vi "GUI_Camera_FFT.vi"() -> ()   [LabVIEW 2020]
uses:
  Shared/GUI_Template/GUI_master/tcp_new_data_event.ctl
  Shared/GUI_Template/GUI_master/tcp new data cluster.ctl
panel:
  out "tcp data event":T1
  in  "Refresh Button":bool
  in  "Select device":string(combo)="PL1-PresCtl"
  in  "stop":bool
  in  "triggermode::1":bool caption="Blank Button"
  in  "exposure::1":dbl=0.001 caption="Exposure" min=0.0001 max=1.0 format="%_4p"
  in  "GUIdevice 1":string="TS-ChromexCam"
  out "image::1":T2(plugin-control) caption="image for joost"
  in  "insert tag":bool=TRUE
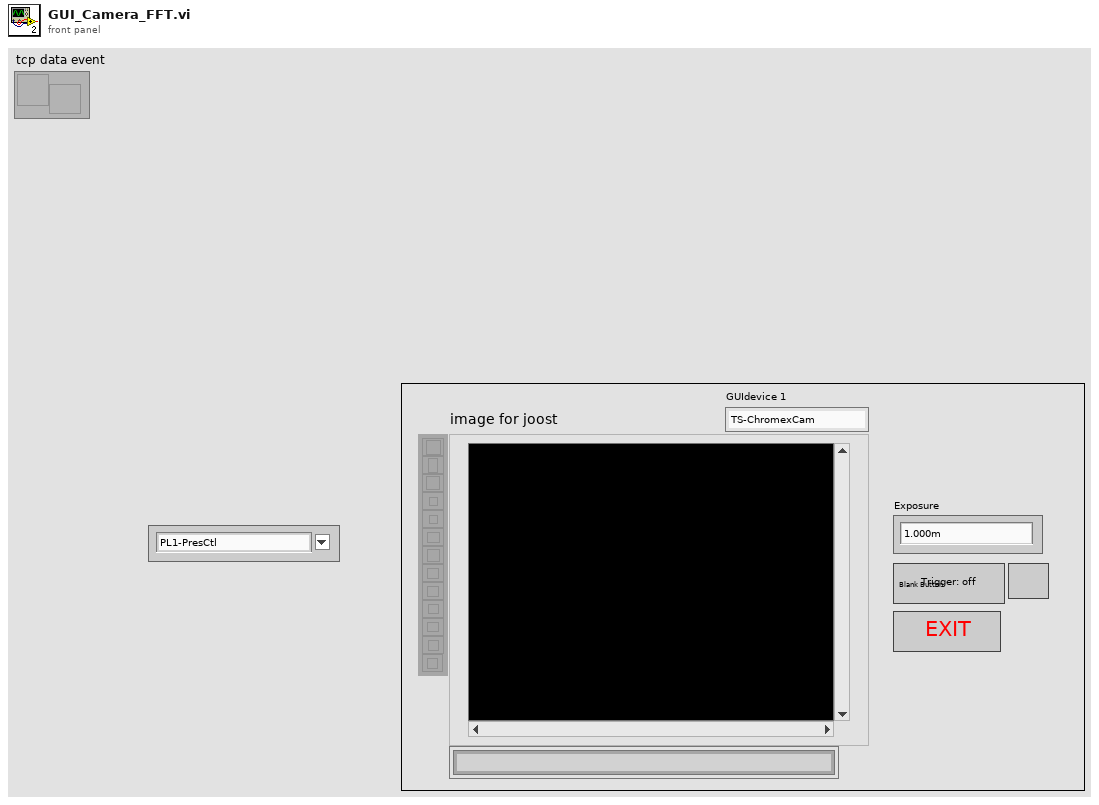
[diagram p1: front panel]
types:
  T1 = typedef "tcp_new_data_event.ctl" = refnum<user-event>
  T2 = typedef "IMAQ Image.ctl" = refnum<image>
  T3 = typedef "Image Type" = u32
  T4 = enum32{"invalid app kind", "Development System", "Run Time System", "Student Edition", "Embedded LabVIEW", "Evaluation", "Custom"}
  T5 = typedef "tcp new data cluster.ctl" = cluster{"EventEnum":enum16{"new data", "connection status update"}, "Device name":string}
  T6 = enum32{"Invalid", "Standard", "Closed", "Hidden", "Minimized", "Maximized"}
  T7 = cluster{"Core":cluster{"Current VI Reference":refnum<vi>, "Close Panel on Exit?":bool}, "Your Boolean data":bool, "Your string data":string, "SuperGUI":cluster{"STOP queue":refnum<queue>, "SuperGUI ref":refnum<vi>}}
  T8 = cluster{"STOP queue":refnum<queue>, "SuperGUI ref":refnum<vi>}
  T9 = cluster{"Current VI Reference":refnum<vi>, "Close Panel on Exit?":bool}
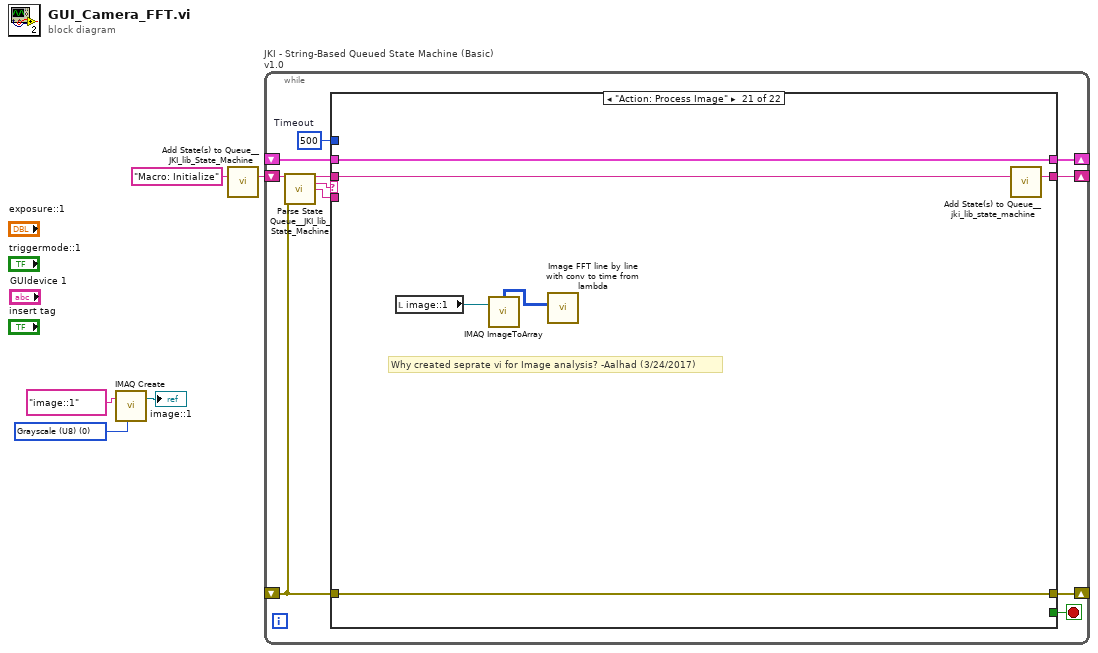
[diagram p0: block diagram]
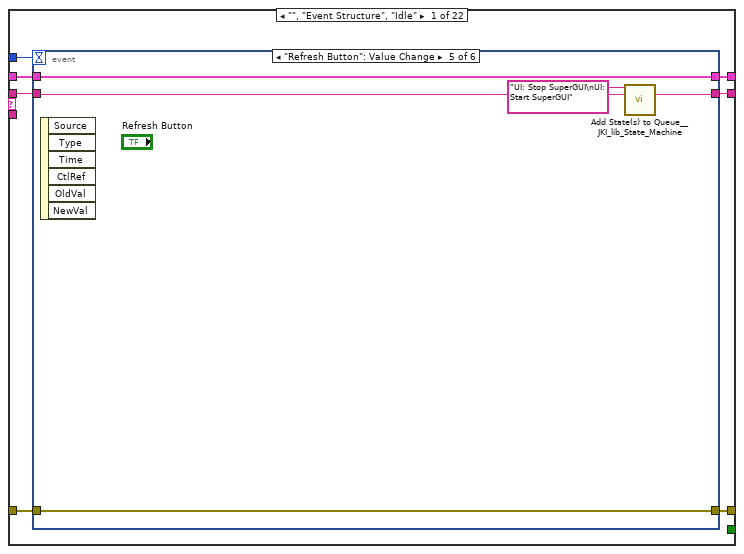
[diagram p2: hidden frame]
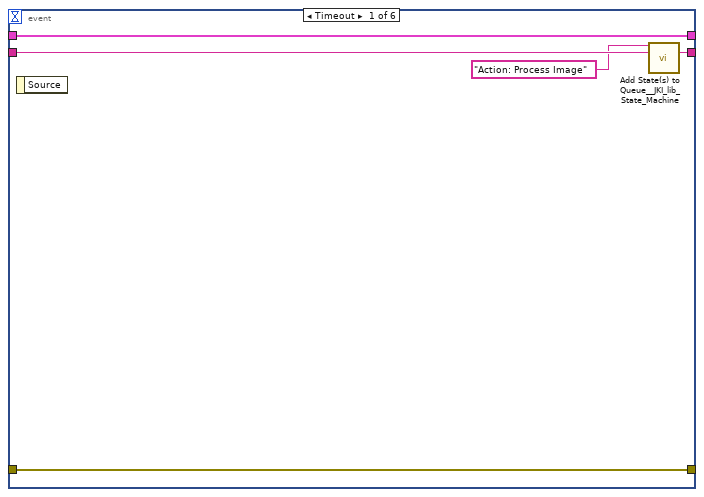
[diagram p3: hidden frame]
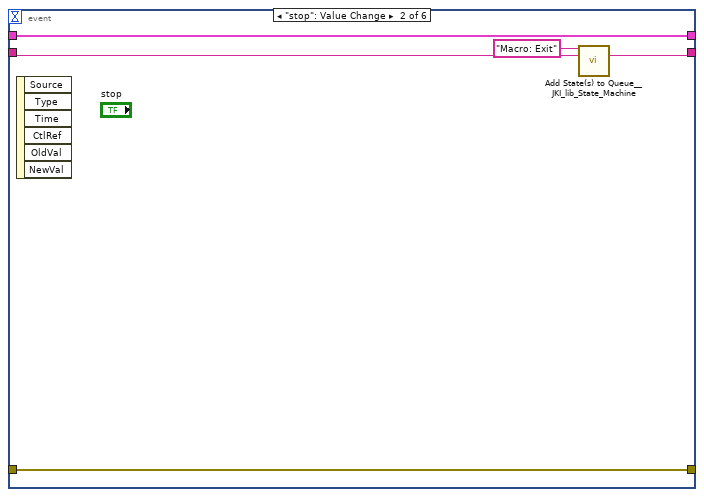
[diagram p4: hidden frame]
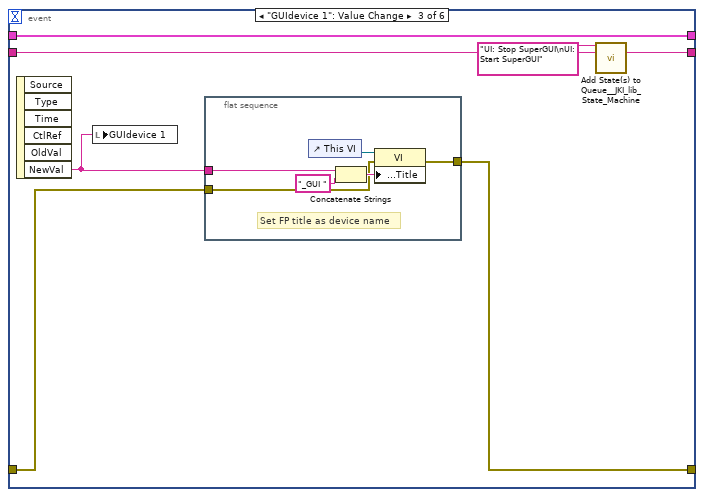
[diagram p5: hidden frame]
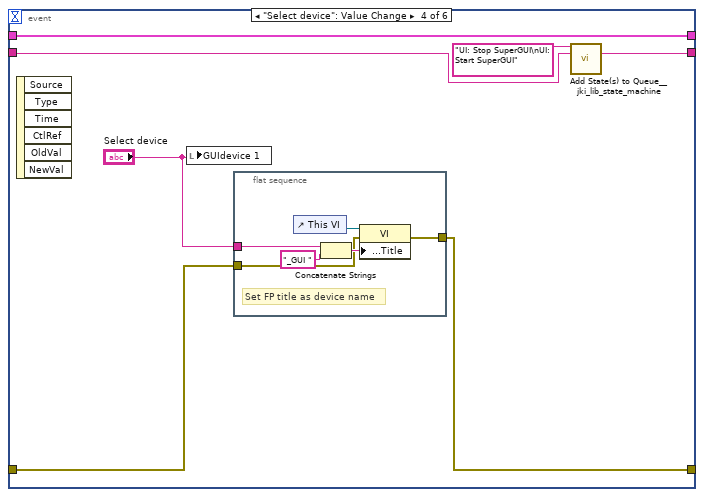
[diagram p6: hidden frame]
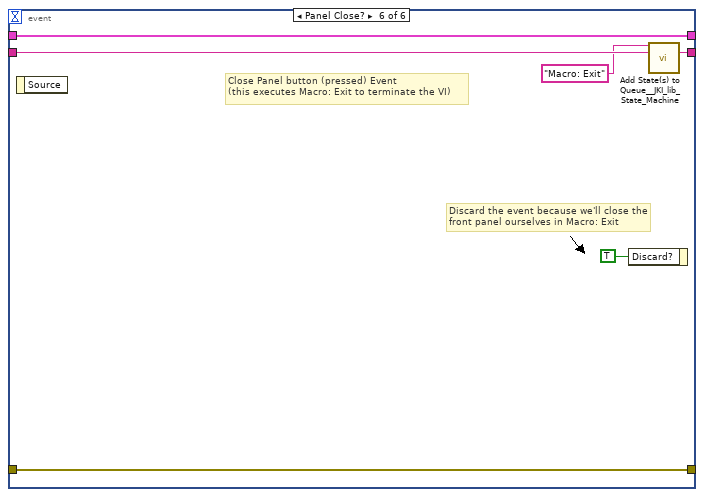
[diagram p7: hidden frame]
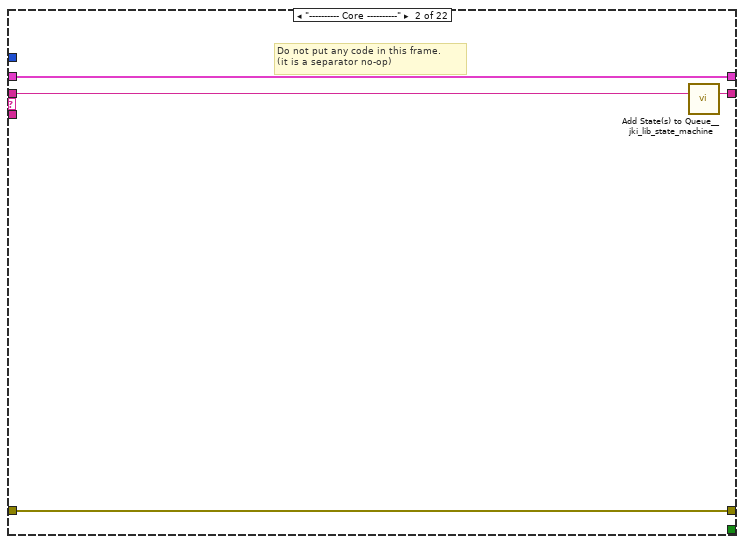
[diagram p8: hidden frame]
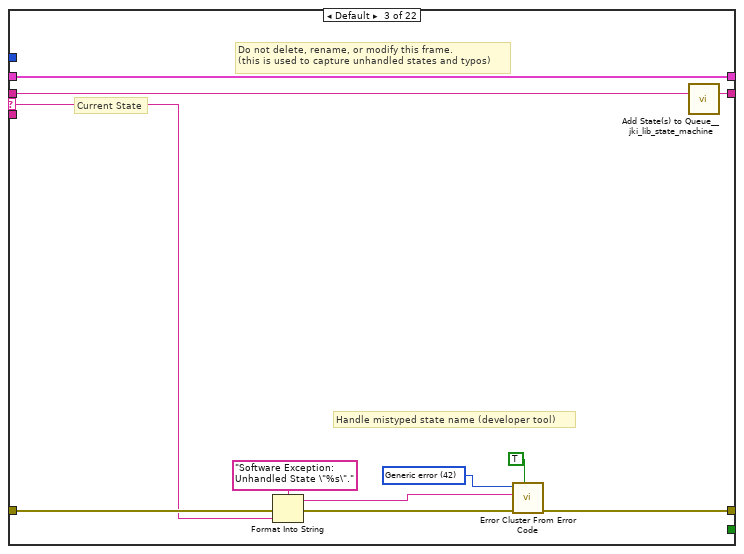
[diagram p9: hidden frame]
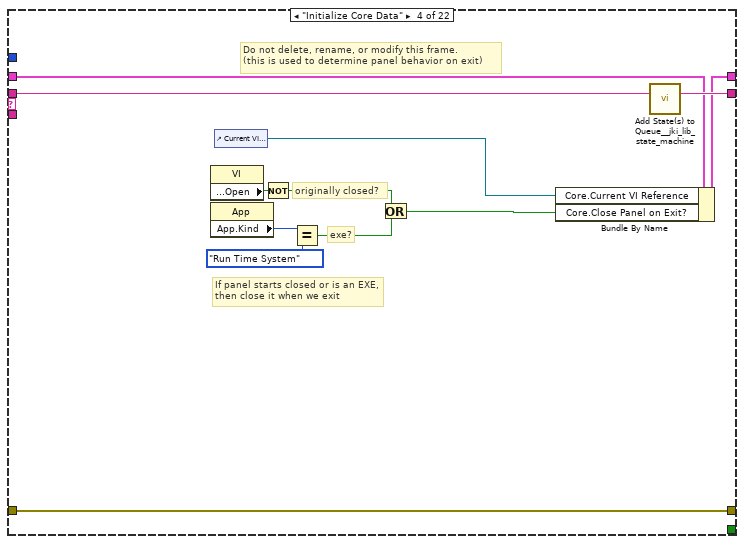
[diagram p10: hidden frame]
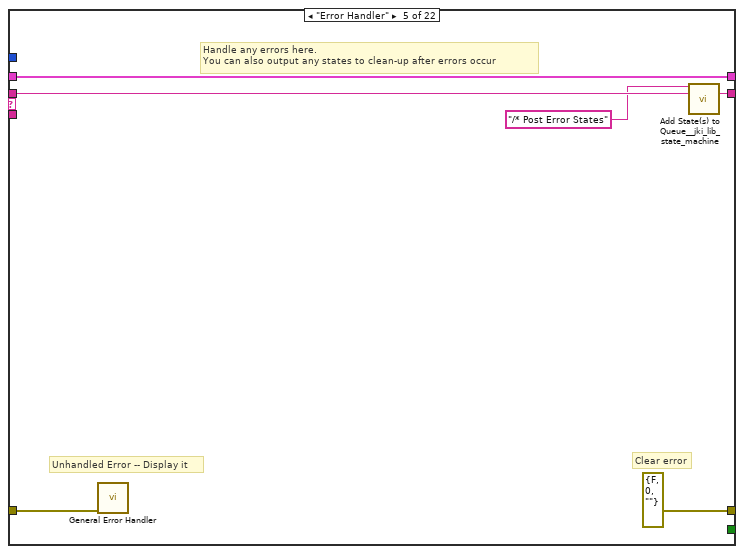
[diagram p11: hidden frame]
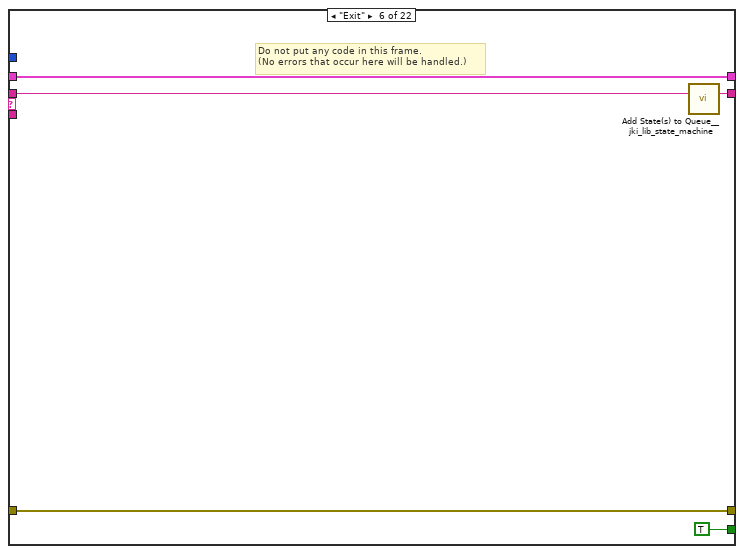
[diagram p12: hidden frame]
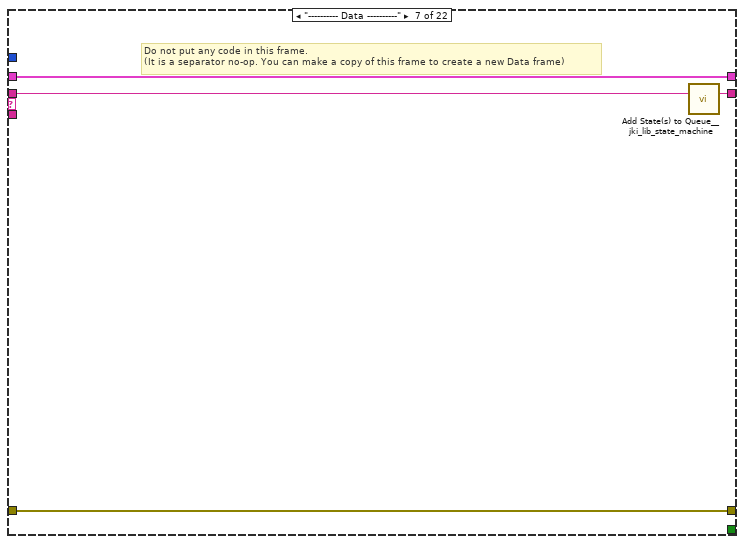
[diagram p13: hidden frame]
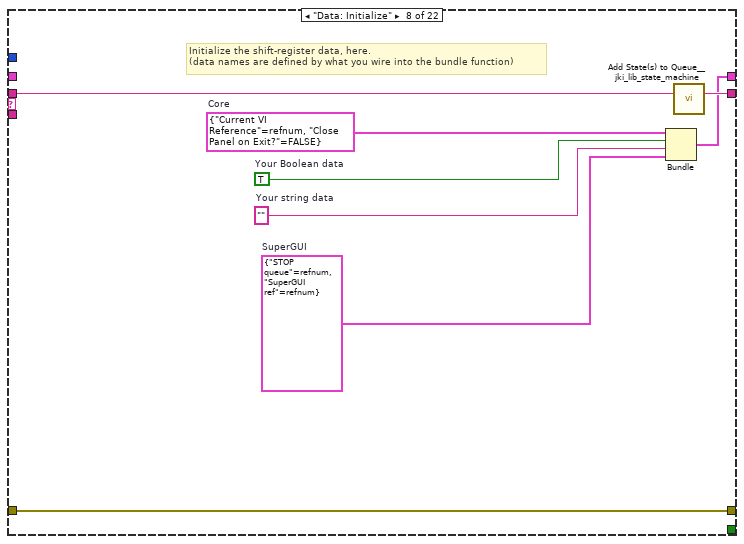
[diagram p14: hidden frame]
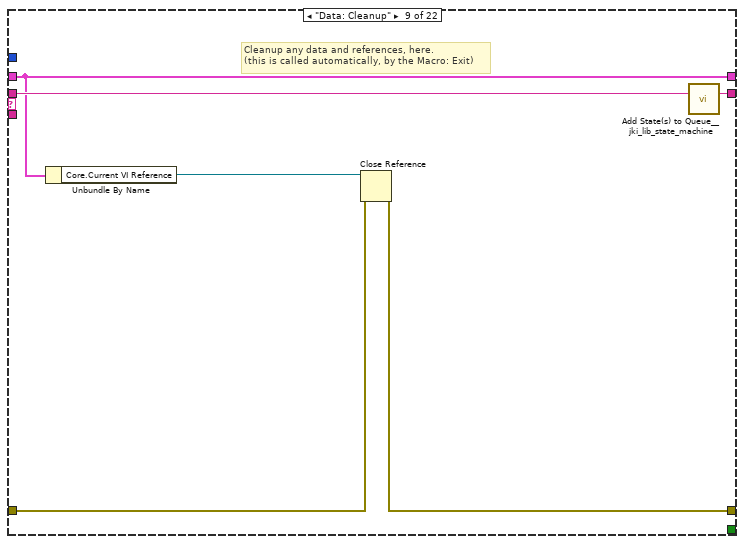
[diagram p15: hidden frame]
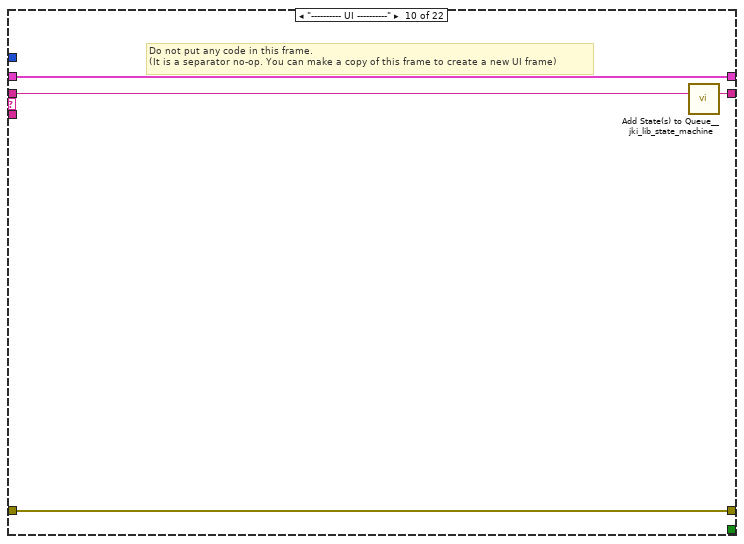
[diagram p16: hidden frame]
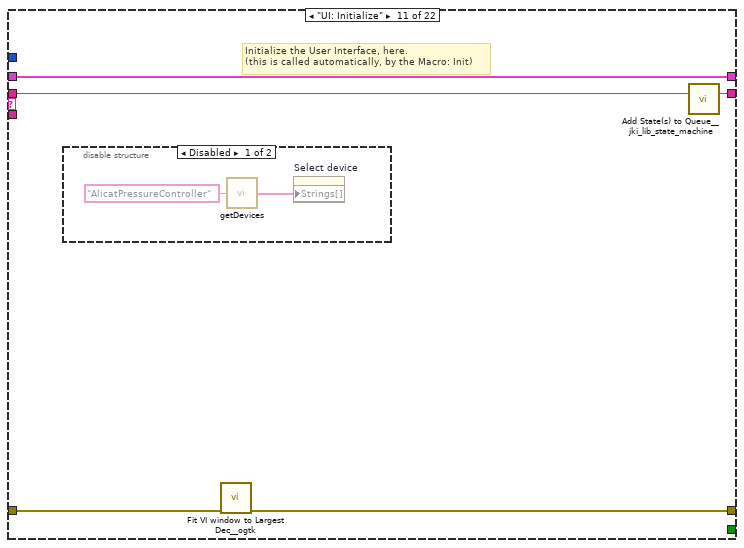
[diagram p17: hidden frame]
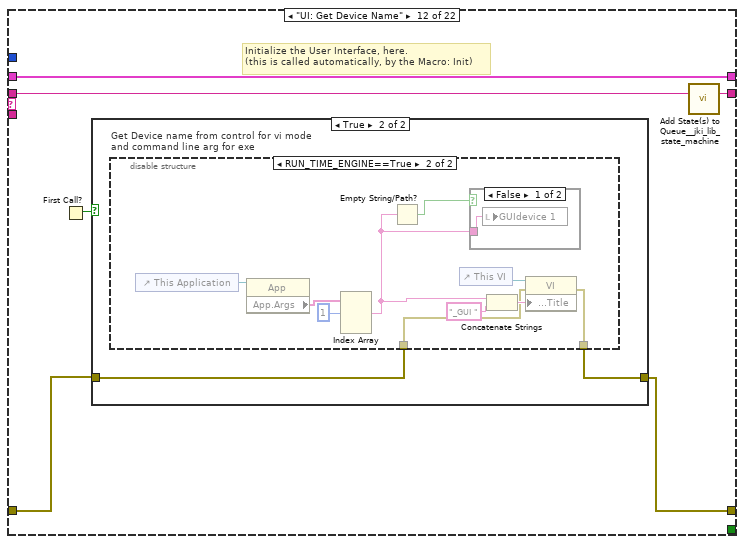
[diagram p19: hidden frame]
diagram:
  w1 = T3 0 items=["Grayscale (U8)", "Grayscale (I16)", "Grayscale (SGL)", "Complex (CSG)", "RGB (U32)", "HSL (U32)", "RGB (U64)", "Grayscale (U16)"] ("Image Type")
  n1 = call "IMAQ Create"("Image Name"="image::1", "Image Type"=w1) -> ("New Image"=→"image::1":T2)  [unwired: 3 in, 1 out]
  n2 = call <vilib>:"Add State(s) to Queue__JKI_lib_State_Machine.vi"("State(s) in (\"\")"="Macro: Initialize") -> ("States Out"=w5:string)  [unwired: 14 in]
  n3 = while "JKI - String-Based Queued State Machine (Basic) v1.0" {
    shift-right: [w9] -> _
    shift-left: _ -> [w8]
    shift-right: [w12] -> _
    shift-left: _ -> [w6]
    shift-right: [w11] -> _
    shift-left: w5 -> [w13]
    stop <- w10 stop-if-true
    w7 = 500  # Timeout
    n4 = call <vilib>:"Parse State Queue__JKI_lib_State_Machine.vi"("State Queue"=w13, "Error In (no error)"=w6) -> ("Remaining States"=w15:string, "Current State"=w16:string, "Arguments"=w14:string)  [unwired: 11 in]
    n5 = case shown="\"Action: Process Image\"" w16 {
      selector: w16 -> [_ _ w75 _ _ _ _ _ _ _ _ _ _ _ _ _ _ _ _ _ _ _]
      tunnel: w15 -> [w23 w74 w79 w97 w103 w108 w112 w120 w126 w130 w135 w143 w178 w186 w192 w203 w229 w234 w244 w248 w254 w258]
      tunnel: w14 -> [_ _ _ _ _ _ _ _ _ _ _ _ _ _ w187 w197 _ _ _ _ _ _]
      tunnel: w8 -> [w21 w71 w77 w88 w100 w106 w109 _ w121 w127 w133 w141 w169 w181 w190 w199 w226 w231 w241 w245 w251 w255]
      tunnel: [w20 w72 w81 w94 errorcluster {"status"=FALSE, "code"=0, "source"=""} ("error out") w105 w110 w117 w122 w128 w131 w138 w162 w179 w188 w200 w227 w232 w242 w246 w252 w256] -> w12
      tunnel: w6 -> [w19 w72 w80 w94 w99 w105 w110 w117 w123 w128 w132 w139 w163 w180 w189 w201 w227 w232 w242 w246 w252 w256]
      tunnel: [w22 w73 w78 w96 w102 w107 w111 w119 w125 w129 w134 w142 w177 w185 w191 w202 w228 w233 w243 w247 w253 w257] -> w11
      tunnel: [_ _ _ _ _ TRUE _ _ _ _ _ _ _ _ _ _ _ _ _ _ _ _] -> w10
      tunnel: [w18 w71 w77 w95 w100 w106 w109 w118 w121 w127 w133 w141 w168 w181 w190 w199 w226 w231 w241 w245 w251 w255] -> w9
      tunnel: w7 -> [w17 _ _ _ _ _ _ _ _ _ _ _ _ _ _ _ _ _ _ _ _ _]
      frame "", "Event Structure", "Idle" {
        n6 = event shown="[4] \"Refresh Button\": Value Change" {
          selector: _ -> [_ _ _ _ _ _]
          dyn-events: _ -> [_ _ _ _ _ _]
          timeout: w17 -> [_ _ _ _ _ _]
          tunnel: w23 -> [w28 w31 w37 w48 w62 w70]
          tunnel: [w27 w30 w36 w47 w61 w69] -> w22
          tunnel: w21 -> [w25 w33 w40 w53 w64 w67]
          tunnel: [w26 w32 w38 w50 w63 w68] -> w20
          tunnel: w19 -> [w26 w32 w39 w51 w63 w68]
          tunnel: [w25 w33 w40 w53 w64 w67] -> w18
          event Timeout {
            n7 = event-data() -> ()  [unwired: 1 in, 1 out]
            n8 = call <vilib>:"Add State(s) to Queue__JKI_lib_State_Machine.vi"("State(s) in Front (\"\")"="Action: Process Image" ("State(s) in Front (\"\")"), "State(s) in (\"\")"=w28) -> ("States Out"=w27:string)  [unwired: 13 in]
          }
          event "stop": Value Change {
            n9 = event-data() -> ()  [unwired: 1 in, 6 out]
            n10 = call <vilib>:"Add State(s) to Queue__JKI_lib_State_Machine.vi"("State(s) in Front (\"\")"="Macro: Exit", "State(s) in (\"\")"=w31) -> ("States Out"=w30:string)  [unwired: 13 in]
          }
          event "GUIdevice 1": Value Change {
            n11 = event-data() -> ("NewVal"=w34:string)  [unwired: 1 in, 5 out]
            n12 = local write "GUIdevice 1"(w34) -> ()
            n13 = flat-sequence {
              tunnel: [w43] -> w38
              tunnel: w39 -> [w42]
              tunnel: w34 -> [w41]
              frame #0 {
                # "Set FP title as device name"
                n14 = control-ref of="This VI"() -> (w46:refnum<vi>)
                n15 = Concatenate Strings(w41, "_GUI ") -> (w45:string)
                n16 = property class="VI"(reference=w46, error in=w42, "Front Panel.Title"=w45) -> (error out=w43:errorcluster)  [unwired: 1 out]
              }
            }
            n17 = call <vilib>:"Add State(s) to Queue__JKI_lib_State_Machine.vi"("State(s) in Front (\"\")"="UI: Stop SuperGUI\nUI: Start SuperGUI", "State(s) in (\"\")"=w37) -> ("States Out"=w36:string)  [unwired: 13 in]
          }
          event "Select device": Value Change {
            n18 = event-data() -> ()  [unwired: 1 in, 6 out]
            n19 = local write "GUIdevice 1"("Select device") -> ()
            n20 = flat-sequence {
              tunnel: [w56] -> w50
              tunnel: w51 -> [w55]
              tunnel: "Select device" -> [w54]
              frame #0 {
                # "Set FP title as device name"
                n21 = control-ref of="This VI"() -> (w59:refnum<vi>)
                n22 = Concatenate Strings(w54, "_GUI ") -> (w58:string)
                n23 = property class="VI"(reference=w59, error in=w55, "Front Panel.Title"=w58) -> (error out=w56:errorcluster)  [unwired: 1 out]
              }
            }
            n24 = call <vilib>:"Add State(s) to Queue__jki_lib_state_machine.vi"("State(s) in Front (\"\")"="UI: Stop SuperGUI\nUI: Start SuperGUI", "State(s) in (\"\")"=w48) -> ("States Out"=w47:string)  [unwired: 13 in]
          }
          event "Refresh Button": Value Change {
            n25 = event-data() -> ()  [unwired: 1 in, 6 out]
            n26 = call <vilib>:"Add State(s) to Queue__JKI_lib_State_Machine.vi"("State(s) in Front (\"\")"="UI: Stop SuperGUI\nUI: Start SuperGUI", "State(s) in (\"\")"=w62) -> ("States Out"=w61:string)  [unwired: 13 in]
          }
          event Panel Close? {
            # "Discard the event because we'll close the front panel ourselves in Macro: Exit"
            # "Close Panel button (pressed) Event\n(this executes Macro: Exit to terminate the VI)"
            n27 = event-data() -> ()  [unwired: 1 in, 1 out]
            n28 = event-data("Discard?"=TRUE) -> ()  [unwired: 1 in, 1 out]
            n29 = call <vilib>:"Add State(s) to Queue__JKI_lib_State_Machine.vi"("State(s) in Front (\"\")"="Macro: Exit", "State(s) in (\"\")"=w70) -> ("States Out"=w69:string)  [unwired: 13 in]
          }
        }
      }
      frame "---------- Core ----------" {
        # "Do not put any code in this frame.\n(it is a separator no-op)"
        n30 = call <vilib>:"Add State(s) to Queue__jki_lib_state_machine.vi"("State(s) in (\"\")"=w74) -> ("States Out"=w73:string)  [unwired: 14 in]
      }
      frame Default {
        w84 = 42 items=["No error", "Argument error", "Memory is full", "Out of zone", "End of file", "File already open", "Generic file I/O error", "File not found", "File permission error", "Disk is full", "Duplicate path", "Too many files open", "System feature not enabled", "Resource file not found", "Cannot add resource", "Resource not found", "Image not found", "Image memory error", "Pen does not exist", "Config type invalid", "Config token not found", "Config parse error", "Config memory error", "Bad external code format", "Bad external code offset", "External code not present", "Null window", "Destroy window error", "Null menu", "Print aborted", "Bad print record", "Print driver error", "Windows error during printing", "Memory error during printing", "Print dialog error", "Generic print error", "Invalid device refnum", "Device not found", "Device parameter error", "Device unit error", "Cannot open device", "Device call aborted", "Generic error", "Cancelled by user", "Object ID too low", "Object ID too high", "Object not in heap", "Unknown heap", "Unknown object (invalid DefProc)", "Unknown object (DefProc not in table)", "Message out of range", "Invalid (null) method", "Unknown message", "Manager call not supported", "Bad address", "Network operation in progress", "Network operation timed out", "Connection is busy", "Network attribute not supported", "Network error", "Address in use", "System out of memory", "Connection aborted", "Connection refused", "Not connected", "Already connected", "Connection closed", "Initialization error (interapplication manager)", "Bad occurrence", "Wait on unbound occurrence handler", "Occurrence queue overflow", "Datalog type conflict", "Unused", "Unrecognized type (interapplication manager)", "Memory corrupt", "Failed to make temporary DLL", "Old CIN version", "Drag socket not found", "Failed to load drop-object", "Failed to register OLE object", "Failed to release OLE object", "Format specifier type mismatch", "Unknown format specifier", "Too few format specifiers", "Too many format specifiers", "Scan failed", "Newer CIN version", "Error converting to variant", "Runtime menu error", "Password tampered", "Variant attribute not found", "Incompatible variant data type", "Event data is not available", "Event Store is not present", "Occurrence is not found", "Event Queue is not created", "Event info is not available", "Refnum passed is NULL", "Error retrieving Class GUID", "Error retrieving CoClass GUID", "Error retrieving TypeLib GUID.", "Bad built application magic bytes.", "Specific driver is different from the specific driver associated with the Logical Name.", "There is no session opened to the class driver.", "Max Error", "MAX - Error with config objects", "MAX - Error loading configuration", "MAX - Group not supported"]
        # "Current State"
        # "Do not delete, rename, or modify this frame.\n(this is used to capture unhandled states and typos)"
        # "Handle mistyped state name (developer tool)"
        n31 = Format Into String(format string="Software Exception: Unhandled State \"%s\"." ("message"), error in=w80, w75) -> (resulting string=w83:string, error out=w82:errorcluster)  [unwired: 1 in]
        n32 = call <vilib>:"Error Cluster From Error Code.vi"("show call chain? (False)"=TRUE, "error in (no error)"=w82, "error message (\"\")"=w83, "error code (0)"=w84) -> ("error out"=w81:errorcluster)  [unwired: 5 in]
        n33 = call <vilib>:"Add State(s) to Queue__jki_lib_state_machine.vi"("State(s) in (\"\")"=w79) -> ("States Out"=w78:string)  [unwired: 14 in]
      }
      frame "Initialize Core Data" {
        # "Do not delete, rename, or modify this frame.\n(this is used to determine panel behavior on exit)"
        # "originally closed?"
        # "exe?"
        # "If panel starts closed or is an EXE, then close it when we exit"
        n34 = property class="VI"() -> ("Front Panel.Open"=w93:bool)  [unwired: 2 in, 2 out]
        n35 = property class="App"() -> ("App.Kind"=w92:T4)  [unwired: 2 in, 2 out]
        n36 = control-ref of="Current VI Reference"() -> (w86:refnum<vi>)
        n37 = Not(x=w93) -> (.not. x?=w90:bool)
        n38 = Equal?(x=w92, y=T4."Run Time System" ("Application:Kind")) -> (x = y?=w89:bool)
        n39 = Or(x=w90, y=w89) -> (x .or. y?=w87:bool)
        n40 = Bundle By Name(cluster=w88, "Core.Current VI Reference"=w86, "Core.Close Panel on Exit?"=w87) -> (w95:T7)
        n41 = call <vilib>:"Add State(s) to Queue__jki_lib_state_machine.vi"("State(s) in (\"\")"=w97) -> ("States Out"=w96:string)  [unwired: 14 in]
      }
      frame "Error Handler" {
        # "Unhandled Error -- Display it"
        # "Handle any errors here.\nYou can also output any states to clean-up after errors occur"
        # "Clear error"
        n42 = call <vilib>:"General Error Handler.vi"("error in (no error)"=w99) -> ()  [unwired: 10 in, 5 out]
        n43 = call <vilib>:"Add State(s) to Queue__jki_lib_state_machine.vi"("State(s) in Front (\"\")"="/* Post Error States", "State(s) in (\"\")"=w103) -> ("States Out"=w102:string)  [unwired: 13 in]
      }
      frame "Exit" {
        # "Do not put any code in this frame.\n(No errors that occur here will be handled.)"
        n44 = call <vilib>:"Add State(s) to Queue__jki_lib_state_machine.vi"("State(s) in (\"\")"=w108) -> ("States Out"=w107:string)  [unwired: 14 in]
      }
      frame "---------- Data ----------" {
        # "Do not put any code in this frame.\n(It is a separator no-op. You can make a copy of this frame to create a new Data frame)"
        n45 = call <vilib>:"Add State(s) to Queue__jki_lib_state_machine.vi"("State(s) in (\"\")"=w112) -> ("States Out"=w111:string)  [unwired: 14 in]
      }
      frame "Data: Initialize" {
        w113 = T8 {"STOP queue"=refnum, "SuperGUI ref"=refnum}  # SuperGUI
        w114 = T9 {"Current VI Reference"=refnum, "Close Panel on Exit?"=FALSE}  # Core
        w116 = TRUE  # Your Boolean data
        w115 = ""  # Your string data
        # "Initialize the shift-register data, here.\n(data names are defined by what you wire into the bundle function)"
        n46 = Bundle("Core"=w114, "Your Boolean data"=w116, "Your string data"=w115, "SuperGUI"=w113) -> (w118:T7)  [unwired: 1 in]
        n47 = call <vilib>:"Add State(s) to Queue__jki_lib_state_machine.vi"("State(s) in (\"\")"=w120) -> ("States Out"=w119:string)  [unwired: 14 in]
      }
      frame "Data: Cleanup" {
        # "Cleanup any data and references, here.\n(this is called automatically, by the Macro: Exit)"
        n48 = Unbundle By Name(w121) -> ("Core.Current VI Reference"=w124:refnum<vi>)
        n49 = Close Reference(reference=w124, error in (no error)=w123) -> (error out=w122:errorcluster)
        n50 = call <vilib>:"Add State(s) to Queue__jki_lib_state_machine.vi"("State(s) in (\"\")"=w126) -> ("States Out"=w125:string)  [unwired: 14 in]
      }
      frame "---------- UI ----------" {
        # "Do not put any code in this frame.\n(It is a separator no-op. You can make a copy of this frame to create a new UI frame)"
        n51 = call <vilib>:"Add State(s) to Queue__jki_lib_state_machine.vi"("State(s) in (\"\")"=w130) -> ("States Out"=w129:string)  [unwired: 14 in]
      }
      frame "UI: Initialize" {
        # "Initialize the User Interface, here.\n(this is called automatically, by the Macro: Init)"
        n52 = disable-structure shown="Disabled" {
          frame Disabled {
            n53 = call "getDevices.vi"("Device Class"="AlicatPressureController") -> ("All Devices"=w136:string[])
            n54 = property on="Select device" class="CmbBox"("Strings[]"=w136) -> ()  [unwired: 2 in, 2 out]
          }
          frame Enabled {
          }
        }
        n55 = call <userlib>:"Fit VI window to Largest Dec__ogtk.vi"("error in (no error)"=w132) -> ("error out"=w131:errorcluster)  [unwired: 5 in, 1 out]
        n56 = call <vilib>:"Add State(s) to Queue__jki_lib_state_machine.vi"("State(s) in (\"\")"=w135) -> ("States Out"=w134:string)  [unwired: 14 in]
      }
      frame "UI: Get Device Name" {
        # "Initialize the User Interface, here.\n(this is called automatically, by the Macro: Init)"
        n57 = First Call?() -> (First Call?: T/F=w140:bool)
        n58 = case shown="True" w140 {
          tunnel: w139 -> [w144 w146]
          tunnel: [w144 w145] -> w138
          frame False {
          }
          frame True {
            n59 = disable-structure "Get Device name from control for vi mode\nand command line arg for exe" shown="RUN_TIME_ENGINE==True" {
              disable-tunnel: w146 -> [w147 w149]
              disable-tunnel: [w147 w148] -> w145
              frame condition #0 (active) {
              }
              frame condition #1 {
                n60 = control-ref of="This Application"() -> (w157:refnum<vi>)
                n61 = property class="App"(reference=w157) -> ("App.Args"=w156:string[])  [unwired: 1 in, 2 out]
                n62 = Index Array(array=w156, index #1=1 ("index")) -> (element #1=w150:string)  [unwired: 2 in, 2 out]
                n63 = Empty String/Path?(string/path=w150) -> (empty?=w154:bool)
                n64 = control-ref of="This VI"() -> (w153:refnum<vi>)
                n65 = case shown="False" w154 {
                  tunnel: w150 -> [w158 _]
                  frame False {
                    n66 = local write "GUIdevice 1"(w158) -> ()
                  }
                  frame True {
                  }
                }
                n67 = Concatenate Strings(w150, "_GUI ") -> (w152:string)
                n68 = property class="VI"(reference=w153, error in=w149, "Front Panel.Title"=w152) -> (error out=w148:errorcluster)  [unwired: 1 out]
              }
            }
          }
        }
        n69 = call <vilib>:"Add State(s) to Queue__jki_lib_state_machine.vi"("State(s) in (\"\")"=w143) -> ("States Out"=w142:string)  [unwired: 14 in]
      }
      frame "UI: Start SuperGUI" {
        # "create stop queue for supergui and its clones"
        # "x100 abort will be dependent on caller VI\nx80 abort will be independent of caller vi, this will abort vi when labview is closed."
        # "Start SuperGUI asynchronous way"
        n70 = vi-ref "GUI_Master_subvi_reentrant_queues.vi"() -> (w161:refnum<vi>)
        n71 = property class="VI"(reference=w161) -> ("Path"=w160:path)  [unwired: 1 in, 2 out]
        n72 = Create User Event(user event datatype=T5 {"EventEnum"=enum."new data", "Device name"="Device name"} ("New Event"), error in=w163) -> (user event=w164:refnum<user-event>, error out=w170:errorcluster)
        "tcp data event" <- w164
        n73 = control-ref of="This Application"() -> (w167:refnum<vi>)
        n74 = control-ref of="This VI"() -> (w166:refnum<vi>)
        n75 = Open VI Reference(type specifier VI Refnum (for type only)=refnum<vi> refnum, vi path=w160, options=256) -> (vi reference=w176:refnum<vi>, error out=w175:errorcluster)  [unwired: 3 in]
        n76 = register-events(w164) -> ()  [unwired: 2 in, 2 out]
        n77 = call "supergui create stop queue.vi"() -> ("STOP Queue out"=w172:refnum<queue>)  [unwired: 11 in]
        n78 = Current VI's Menubar() -> (w165:refnum<k9>)
        n79 = call-by-ref "Start Asynchronous Call"(reference=w176, error in=w175, "STOP Queue in"=w172, "This Application"=w167, 8:"error in (no error)"=w170, "tcp data event"=w164, "Caller menu reference"=w165, "Caller VI ref"=w166) -> (reference out=w159:refnum<vi>, error out=w162:errorcluster)  [unwired: 5 in, 1 out]
        n80 = Bundle By Name(cluster=w169, "SuperGUI.SuperGUI ref"=w159, "SuperGUI.STOP queue"=w172) -> (w168:T7)
        n81 = call <vilib>:"Add State(s) to Queue__jki_lib_state_machine.vi"("State(s) in (\"\")"=w178) -> ("States Out"=w177:string)  [unwired: 14 in]
      }
      frame "UI: Stop SuperGUI" {
        # "Stop Supergui Clone and wait until it exit properly"
        n82 = Unbundle By Name(w181) -> ("SuperGUI.SuperGUI ref"=w183:refnum<vi>, "SuperGUI.STOP queue"=w182:refnum<queue>)
        n83 = Release Queue(queue=w182, error in (no error)=w180) -> (error out=w184:errorcluster)  [unwired: 1 in, 2 out]
        n84 = call-by-ref "Wait On Asynchronous Call"(reference=w183, error in=w184) -> ("error out"=w179:errorcluster)  [unwired: 11 in, 2 out]
        n85 = call <vilib>:"Add State(s) to Queue__jki_lib_state_machine.vi"("State(s) in (\"\")"=w186) -> ("States Out"=w185:string)  [unwired: 14 in]
      }
      frame "UI: Cursor Set" {
        # "Argument"
        # "Set and Unset Cursor Busy.\n(Usage: \"UI: Cursor Set >> Busy|Idle\")"
        n86 = case shown="\"Idle\", Default" w187 {
          tunnel: w189 -> [w194 w196]
          tunnel: [w193 w195] -> w188
          frame "Idle", Default {
            n87 = call <vilib>:"Unset Busy.vi"("error in (no error)"=w194) -> ("error out"=w193:errorcluster)  [unwired: 10 in]
          }
          frame "Busy" {
            n88 = call <vilib>:"Set Busy.vi"("error in (no error)"=w196) -> ("error out"=w195:errorcluster)  [unwired: 9 in, 1 out]
          }
        }
        n89 = call <vilib>:"Add State(s) to Queue__jki_lib_state_machine.vi"("State(s) in (\"\")"=w192) -> ("States Out"=w191:string)  [unwired: 14 in]
      }
      frame "UI: Front Panel State" {
        # "Argument"
        # "Set Front Panel Open or Closed\n(Usage: \"UI: Front Panel State >> Open|Close\")"
        n90 = Unbundle By Name(w199) -> ("Core.Current VI Reference"=w198:refnum<vi>)
        n91 = case shown="\"Open\", Default" w197 {
          tunnel: w201 -> [w207 w220]
          tunnel: [w209 w221] -> w200
          tunnel: w198 -> [w208 w218]
          frame "Open", Default {
            n92 = property class="VI"(reference=w208, error in=w207) -> (reference out=w205:refnum<vi>, error out=w206:errorcluster, "Front Panel.Open"=w204:bool)
            n93 = case shown="False" w204 {
              tunnel: [w212 w215] -> w209
              tunnel: w206 -> [w211 w215]
              tunnel: w205 -> [w210 _]
              frame False {
                n94 = invoke class="VI" method="FP.Open"(reference=w210, error in=w211, "Activate"=TRUE, "State"=T6."Standard") -> (error out=w212:errorcluster)  [unwired: 1 in, 4 out]
              }
              frame True {
              }
            }
          }
          frame "Close" {
            n95 = property class="VI"(reference=w218, error in=w220) -> (reference out=w217:refnum<vi>, error out=w219:errorcluster, "Front Panel.Open"=w216:bool)
            n96 = case shown="True" w216 {
              tunnel: [w222 w225] -> w221
              tunnel: w219 -> [w222 w224]
              tunnel: w217 -> [_ w223]
              frame False {
              }
              frame True {
                n97 = invoke class="VI" method="FP.Close"(reference=w223, error in=w224) -> (error out=w225:errorcluster)  [unwired: 1 in, 2 out]
              }
            }
          }
        }
        n98 = call <vilib>:"Add State(s) to Queue__jki_lib_state_machine.vi"("State(s) in (\"\")"=w203) -> ("States Out"=w202:string)  [unwired: 14 in]
      }
      frame "---------- Macro ----------" {
        # "Do not put any code in this frame.\n(It is a separator no-op. You can make a copy of this frame to create a new Macro frame)"
        n99 = call <vilib>:"Add State(s) to Queue__jki_lib_state_machine.vi"("State(s) in (\"\")"=w229) -> ("States Out"=w228:string)  [unwired: 14 in]
      }
      frame "Macro: Initialize" {
        # "Initialization Macro\n(This is called once, when the VI starts)"
        n100 = call <vilib>:"Add State(s) to Queue__jki_lib_state_machine.vi"("State(s) in Front (\"\")"="Data: Initialize\nInitialize Core Data\nUI: Initialize\nUI: Get Device Name\nUI: Start SuperGUI\nUI: Front Panel State >> Open", "State(s) in (\"\")"=w234) -> ("States Out"=w233:string)  [unwired: 13 in]
      }
      frame "Macro: Exit" {
        # "Exit Macro\n(This is called once, when the VI exits)"
        n101 = Unbundle By Name(w241) -> ("Core.Close Panel on Exit?"=w240:bool)
        n102 = Select(t="UI: Front Panel State >> Close", s=w240, f="") -> (s? t:f=w237:string)
        n103 = call <vilib>:"Add State(s) to Queue__jki_lib_state_machine.vi"("State(s) in (\"\")"=w237, "State(s) at Back (\"\")"="Data: Cleanup\nExit") -> ("States Out"=w235:string)  [unwired: 13 in]
        n104 = call <vilib>:"Add State(s) to Queue__jki_lib_state_machine.vi"("State(s) in Front (\"\")"=w235, "State(s) in (\"\")"=w244) -> ("States Out"=w243:string)  [unwired: 13 in]
      }
      frame "---------- New Category ----------" {
        # "Template Separator\n(You can make a copy of, or modify, this frame)"
        n105 = call <vilib>:"Add State(s) to Queue__jki_lib_state_machine.vi"("State(s) in (\"\")"=w248) -> ("States Out"=w247:string)  [unwired: 14 in]
      }
      frame "Action: Process Image" {
        # "Why created seprate vi for Image analysis? -Aalhad (3/24/2017)"
        n106 = local read "image::1"() -> (w250:T2)
        n107 = call "IMAQ ImageToArray"("Image"=w250) -> ("Image Pixels (U8)"=w249:u8[][])  [unwired: 3 in, 4 out]
        n108 = call "Image FFT line by line with conv to time from lambda.vi"("Input image 2"=w249) -> ()  [unwired: 11 in]
        n109 = call <vilib>:"Add State(s) to Queue__jki_lib_state_machine.vi"("State(s) in (\"\")"=w254) -> ("States Out"=w253:string)  [unwired: 14 in]
      }
      frame "New Category: 2" {
        # "Your code here.\n(You can make a copy of, or modify, this frame)"
        n110 = call <vilib>:"Add State(s) to Queue__jki_lib_state_machine.vi"("State(s) in (\"\")"=w258) -> ("States Out"=w257:string)  [unwired: 14 in]
      }
    }
  }
